vi "Symmetrize.vi"   [LabVIEW 2016, in "xy_utilities.lvlib"]
doc: "Compute the Symmetric and Antisymmetric functions.\n\nWire data to the data input to determine the polymorphic instance to use or manually select the instance."
uses:
  xy_utilities.lvlib
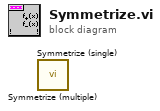
[diagram p0: block diagram]
diagram:
  n1 = call "Symmetrize (multiple).vi"() -> ()  [unwired: 8 in, 4 out]
  n2 = call "Symmetrize (single).vi"() -> ()  [unwired: 8 in, 4 out]
